vi "CSTK_Enum_Creator_Dialog.vi"(0 "Enable":bool=TRUE caption="启用", 1 "标签名输入":string, 2 "样式输入":u32=3062, 3 "项名输入":string, 4 "新建？":bool, 5 "error in (no error)":errorcluster caption="错误输入（无错误）") -> (15 "标签名输出":string, 16 "样式输出":u32, 17 "项名输出":string, 18 "确定":bool, 19 "error out":errorcluster caption="错误输出")   [LabVIEW 2015, in "CSTK_Enum Creator.lvlib"]
doc: "显示标准对话框，提示用户输入用户名、密码等信息。\n--------------------\n\n该Express VI配置如下:\n\n显示给用户的信息:请输入注释\n该输入为:"
uses:
  CSTK_Enum Creator.lvlib
  <userlib>/_OpenG.lib/array/array.llb/Remove Duplicates from 1D Array (String)__ogtk.vi
  user32.dll
panel:
  in  "标签名":string
  in  "样式":u32(ring)=3062 items=["枚举（经典）"=3023, "枚举（系统）"=3062, "枚举（新式）"=21605]
  in  "项名":string
  in  "Cancel":bool caption="取消"
  in  "OK":bool caption="OK2"
  # "Enum Creator"
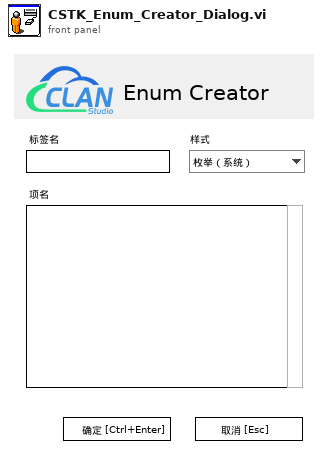
[diagram p1: front panel]
types:
  T1 = enum8{"Enabled", "Disabled", "Disabled and Grayed Out"}
  T2 = enum32{"Invalid", "Standard", "Closed", "Hidden", "Minimized", "Maximized"}
  T3 = typedef "eventvkey.ctl" = enum16{"ASCII", "Enter", "Return", "Shift", "Ctrl", "Alt", "Cmd", "Opt", "Caps", "NumLock", "Clear", "Break", "Up", "Down", "Left", "Right", "Insert", "Delete", "Home", "End", "PageUp", "PageDown", "Escape", "Help", "Pause", "ScrollLock", "F1", "F2", "F3", "F4", "F5", "F6", "F7", "F8", "F9", "F10", "F11", "F12", "F13", "F14", "F15", "F16", "F17", "F18", "F19", "F20", "F21", "F22", "F23", "F24", "Play", "VolumeUp", "VolumeDown", "Mute", "Two Byte Char"}
  T4 = cluster{"Shift":bool, "Ctrl":bool, "Alt":bool, "Cmd":bool, "Opt":bool}
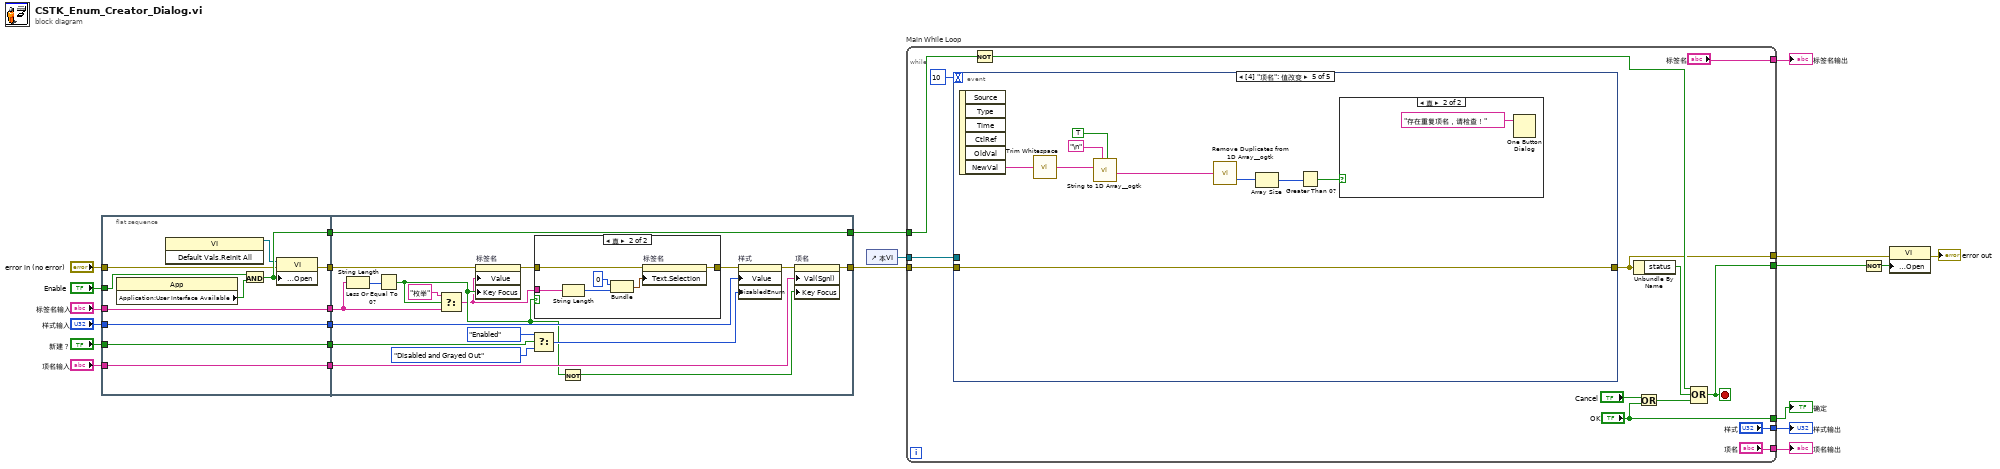
[diagram p0: block diagram]
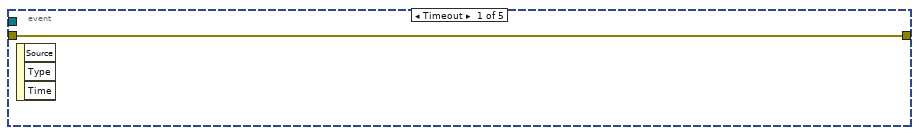
[diagram p3: hidden frame]
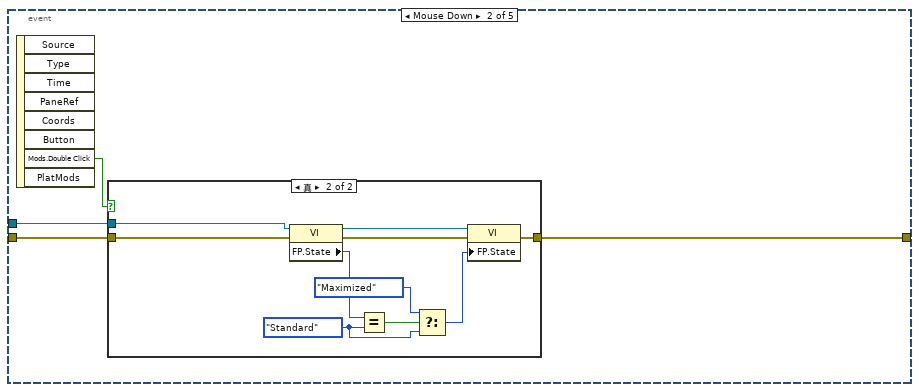
[diagram p4: hidden frame]
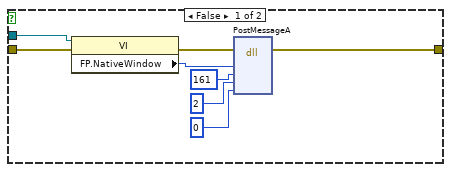
[diagram p5: hidden frame]
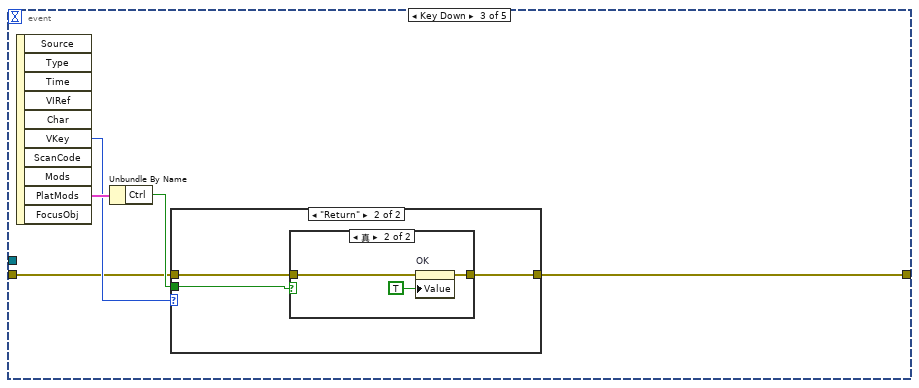
[diagram p6: hidden frame]
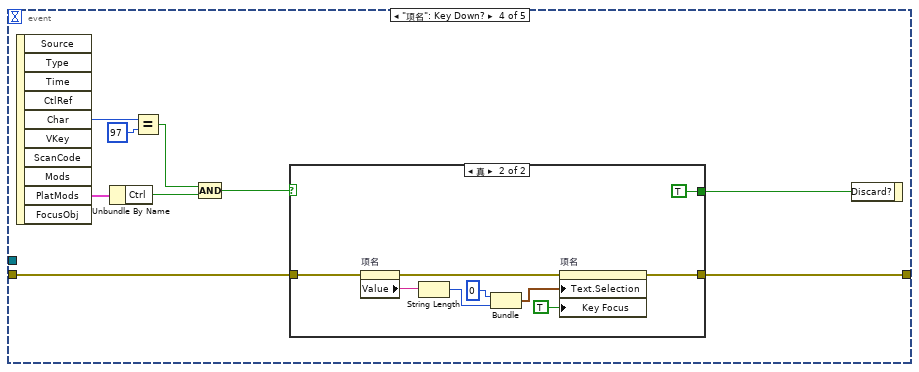
[diagram p9: hidden frame]
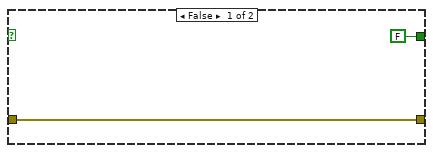
[diagram p10: hidden frame]
diagram:
  n1 = flat-sequence {
    tunnel: [w33] -> w16
    tunnel: [w31] -> w15
    tunnel: "error in (no error)" -> [w28]
    tunnel: "Enable" -> [w32]
    tunnel: [w27] -> w12
    tunnel: "标签名输入" -> [w27]
    tunnel: [w26] -> w10
    tunnel: "样式输入" -> [w26]
    tunnel: [w25] -> w8
    tunnel: "项名输入" -> [w25]
    tunnel: "新建？" -> [w24]
    tunnel: [w24] -> w2
    tunnel: [w51] -> w17
    tunnel: [w46] -> w21
    tunnel: w16 -> [w47]
    tunnel: w15 -> [w51]
    tunnel: w12 -> [w39]
    tunnel: w10 -> [w50]
    tunnel: w8 -> [w49]
    tunnel: w2 -> [w42]
    frame #0 {
      n2 = property class="App"() -> ("Application:User Interface Available"=w30:bool)  [unwired: 2 in, 2 out]
      n3 = invoke class="VI" method="Default Vals.Reinit All"() -> (reference out=w29:refnum<vi>)  [unwired: 3 in, 2 out]
      n4 = And(x=w32, y=w30) -> (x .and. y?=w31:bool)
      n5 = property class="VI"(reference=w29, error in=w28, "Front Panel Window:Open"=w31) -> (error out=w33:errorcluster)  [unwired: 1 out]
    }
    frame #1 {
      n6 = String Length(string=w39) -> (length=w41:i32)
      n7 = Less Or Equal To 0?(x=w41) -> (x <= 0?=w38:bool)
      n8 = Select(t="枚举", s=w38, f=w39) -> (s? t:f=w34:string)
      n9 = property on="标签名" class="Str"(error in=w47, "Value"=w34, "Key Focus"=w38) -> (error out=w36:errorcluster)  [unwired: 1 in, 1 out]
      n10 = Select(t=T1."Enabled" ("禁用"), s=w42, f=T1."Disabled and Grayed Out" ("禁用")) -> (s? t:f=w45:T1)
      n11 = case shown="真" w38 {
        tunnel: [w52 w57] -> w37
        tunnel: w36 -> [w52 w58]
        tunnel: w34 -> [_ w55]
        frame False {
        }
        frame True {
          n12 = String Length(string=w55) -> (length=w54:i32)
          n13 = Bundle("Selection Start"=u32 0, w54) -> (w53:cluster{"Selection Start":u32, i32})  [unwired: 1 in]
          n14 = property on="标签名" class="Str"(error in=w58, "Text.Selection"=w53) -> (error out=w57:errorcluster)  [unwired: 1 in, 1 out]
        }
      }
      n15 = Not(x=w38) -> (.not. x?=w35:bool)
      n16 = property on="样式" class="Ring (严格)"(error in=w37, "Value"=w50, "DisabledEnum"=w45) -> (error out=w48:errorcluster)  [unwired: 1 in, 1 out]
      n17 = property on="项名" class="Str"(error in=w48, "Val(Sgnl)"=w49, "Key Focus"=w35) -> (error out=w46:errorcluster)  [unwired: 1 in, 1 out]
    }
  }
  n18 = control-ref of="本VI"() -> (w1:refnum<vi>)
  n19 = while "Main While Loop" {
    tunnel: ["OK"] -> w13
    tunnel: w17 -> [w71]
    tunnel: [w69] -> w22
    tunnel: w21 -> [w64]
    tunnel: [w63] -> w20
    tunnel: ["样式"] -> w6
    tunnel: ["标签名"] -> w5
    tunnel: ["项名"] -> w4
    tunnel: w1 -> [w59]
    stop <- w69 stop-if-true
    n20 = event shown="[4] \"项名\": 值改变" {
      selector: _ -> [_ _ _ _ _]
      dyn-events: _ -> [_ _ _ _ _]
      timeout: 10 -> [_ _ _ _ _]
      tunnel: w64 -> [w73 w76 w97 w116 w131]
      tunnel: [w73 w75 w96 w117 w131] -> w63
      tunnel: w59 -> [_ w77 _ _ _]
      event Timeout {
        n21 = event-data() -> ()  [unwired: 1 in, 3 out]
      }
      event Mouse Down {
        n22 = event-data() -> ("Mods.Double Click"=w74:bool)  [unwired: 1 in, 7 out]
        n23 = case shown="真" w74 {
          tunnel: w77 -> [w80 w88]
          tunnel: w76 -> [w79 w87]
          tunnel: [w78 w86] -> w75
          frame False {
            n24 = property class="VI"(reference=w80, error in=w79) -> (error out=w81:errorcluster, "FP.NativeWindow"=w82:u64)  [unwired: 1 out]
            n25 = dll-call lib="user32.dll" fn="PostMessageA"(error in=w81, "hWnd"=w82, "Msg"=161, "wParam"=2, "IParam"=0 ("wParam")) -> (error out=w78:errorcluster)  [unwired: 7 in, 1 out]
          }
          frame True {
            w92 = T2."Standard" ("Front Panel Window:State")
            n26 = property class="VI"(reference=w88, error in=w87) -> (reference out=w93:refnum<vi>, error out=w94:errorcluster, "FP.State"=w89:T2)
            n27 = Equal?(x=w89, y=w92) -> (x = y?=w90:bool)
            n28 = Select(t=T2."Maximized" ("Front Panel Window:State"), s=w90, f=w92) -> (s? t:f=w95:T2)
            n29 = property class="VI"(reference=w93, error in=w94, "FP.State"=w95) -> (error out=w86:errorcluster)  [unwired: 1 out]
          }
        }
      }
      event Key Down {
        n30 = event-data() -> ("VKey"=w99:T3, "PlatMods"=w100:T4)  [unwired: 1 in, 8 out]
        n31 = Unbundle By Name(w100) -> ("Ctrl"=w98:bool)
        n32 = case shown="\"Return\"" w99 {
          tunnel: w98 -> [_ w104]
          tunnel: w97 -> [w101 w103]
          tunnel: [w101 w102] -> w96
          frame "ASCII", Default {
          }
          frame "Return" {
            n33 = case shown="真" w104 {
              tunnel: w103 -> [w105 w107]
              tunnel: [w105 w106] -> w102
              frame False {
              }
              frame True {
                n34 = property on="OK" class="Bool (严格)"(error in=w107, "Value"=TRUE ("OK")) -> (error out=w106:errorcluster)  [unwired: 1 in, 1 out]
              }
            }
          }
        }
      }
      event "项名": Key Down? {
        n35 = event-data() -> ("Char"=w110:i16, "PlatMods"=w115:T4)  [unwired: 1 in, 8 out]
        n36 = Unbundle By Name(w115) -> ("Ctrl"=w111:bool)
        n37 = Equal?(x=w110, y=i16 97) -> (x = y?=w113:bool)
        n38 = Compound Arithmetic op=AND ("复合运算")(w113, w111) -> (w112:bool)
        n39 = case shown="真" w112 {
          tunnel: [w119 w123] -> w117
          tunnel: w116 -> [w119 w128]
          tunnel: [FALSE TRUE] -> w109
          frame False {
          }
          frame True {
            n40 = property on="项名" class="Str"(error in=w128) -> (error out=w127:errorcluster, "Value"=w121:string)  [unwired: 1 in, 1 out]
            n41 = String Length(string=w121) -> (length=w125:i32)
            n42 = Bundle(0, w125) -> (w124:cluster{i32, i32})  [unwired: 1 in]
            n43 = property on="项名" class="Str"(error in=w127, "Text.Selection"=w124, "Key Focus"=TRUE ("键选中")) -> (error out=w123:errorcluster)  [unwired: 1 in, 1 out]
          }
        }
        n44 = event-data("Discard?"=w109) -> ()  [unwired: 1 in, 1 out]
      }
      event "项名": Value Change {
        n45 = event-data() -> ("NewVal"=w129:string)  [unwired: 1 in, 5 out]
        n46 = call <vilib>:"Trim Whitespace.vi"("string"=w129) -> ("trimmed string"=w137:string)  [unwired: 1 in]
        n47 = call <userlib>:"String to 1D Array__ogtk.vi"("ignore duplicate delimiters? (F=No)"=TRUE, "delimiter (Tab)"="\n", "string"=w137) -> ("Array of Strings"=w134:string[])  [unwired: 8 in]
        n48 = call-poly <userlib>:"Remove Duplicates from 1D Array__ogtk.vi"("Input Array"=w134) -> ("indices of removed elements"=w133:i32[])  [unwired: 1 out]
        n49 = Array Size(array=w133) -> (size(s)=w132:i32)
        n50 = Greater Than 0?(x=w132) -> (x > 0?=w130:bool)
        n51 = case shown="真" w130 {
          frame False {
          }
          frame True {
            n52 = One Button Dialog(message="存在重复项名，请检查！" ("消息")) -> ()  [unwired: 1 in, 1 out]
          }
        }
      }
    }
    n53 = Not(x=w71) -> (.not. x?=w70:bool)
    n54 = Unbundle By Name(w63) -> ("status"=w67:bool)
    n55 = Or(x="Cancel", y="OK") -> (x .or. y?=w68:bool)
    n56 = Compound Arithmetic op=OR(w70, w67, w68) -> (w69:bool)
  }
  "确定" <- w13
  "样式输出" <- w6
  "标签名输出" <- w5
  "项名输出" <- w4
  n57 = Not(x=w22) -> (.not. x?=w23:bool)
  n58 = property class="VI"(error in=w20, "Front Panel Window:Open"=w23) -> (error out=→"error out":errorcluster)  [unwired: 1 in, 1 out]
